vi "Banana_Equal Type Comparison.vi"(6 "verbose? (F)":bool, 7 "Not? (F)":bool, 8 "error in (no error)":errorcluster, 9 "Y":variant, 10 "X":variant) -> (0 "error out":errorcluster, 2 "Equal Types?":bool, 3 "Verbose output":string)   [LabVIEW 2021, in "Bananas.lvlib"]
uses:
  Bananas.lvlib
  <vilib>/Utility/VariantDataType/Type.ctl
  <vilib>/Utility/VariantDataType/VariantType.lvlib
  <vilib>/Utility/Data Type/NI_Data Type.lvlib
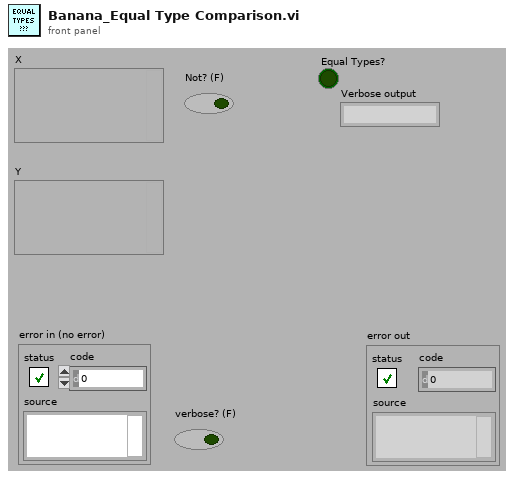
[diagram p1: front panel]
types:
  T1 = typedef "NI_Data Type.lvlib/Data Type.ctl" = enum8{"Invalid Type", "Void", "I8", "I16", "I32", "I64", "U8", "U16", "U32", "U64", "Single Float", "Double Float", "Extended Float", "Single Complex", "Double Complex", "Extended Complex", "Enum U8", "Enum U16", "Enum U32", "Enum U64", "Single Float With Unit", "Double Float With Unit", "Extended Float With Unit", "Single Complex with Unit", "Double Complex with Unit", "Extended Complex with Unit", "Boolean", "String", "Path", "Picture", "Tag", "Array", "Cluster", "Variant", "LV Variant", "Waveform", "Timestamp", "Digital Waveform", "Digital Data", "ExpressData", "Refnum", "External Data", "VI", "Poly VI", "LabVIEW Class Instance", "Fixed Point", "Set Collection", "Map Collection"}
  T2 = typedef "VariantType.lvlib/Type.ctl" = enum8{"Invalid Type", "Void", "I8", "I16", "I32", "I64", "U8", "U16", "U32", "U64", "Single Float", "Double Float", "Extended Float", "Single Complex", "Double Complex", "Extended Complex", "Enum U8", "Enum U16", "Enum U32", "Enum U64", "Single Float With Unit", "Double Float With Unit", "Extended Float With Unit", "Single Complex with Unit", "Double Complex with Unit", "Extended Complex with Unit", "Boolean", "String", "Path", "Picture", "Tag", "Array", "Cluster", "Variant", "LV Variant", "Waveform", "Timestamp", "Digital Waveform", "Digital Data", "ExpressData", "Refnum", "External Data", "VI", "Poly VI", "LabVIEW Class Instance", "Fixed Point"}
  T3 = typedef "NI_Data Type.lvlib/Refnum Type.ctl" = enum16{"NotARefnum", "UnknownRefnum", "Generic", "Datalog", "ByteStream", "Device", "Occurence", "TCPNetConnection", "Auto", "Menu", "Imaq", "Hardware", "DataSocket", "Visa", "IVI", "UDPNetConnection", "Notifier", "Queue", "Irda", "EventReg", "DotNet", "UserEvent", "Callback", "UNUSED_EMPTY_POSITION", "BlueToothNetConnection", "LVObjApp", "LVObjVI", "LVObjUnknown", "GenericClass", "UserDefinedRefnumTag", "DataValue", "RT FIFO", "TDMS File", "PythonSessionRefnum"}
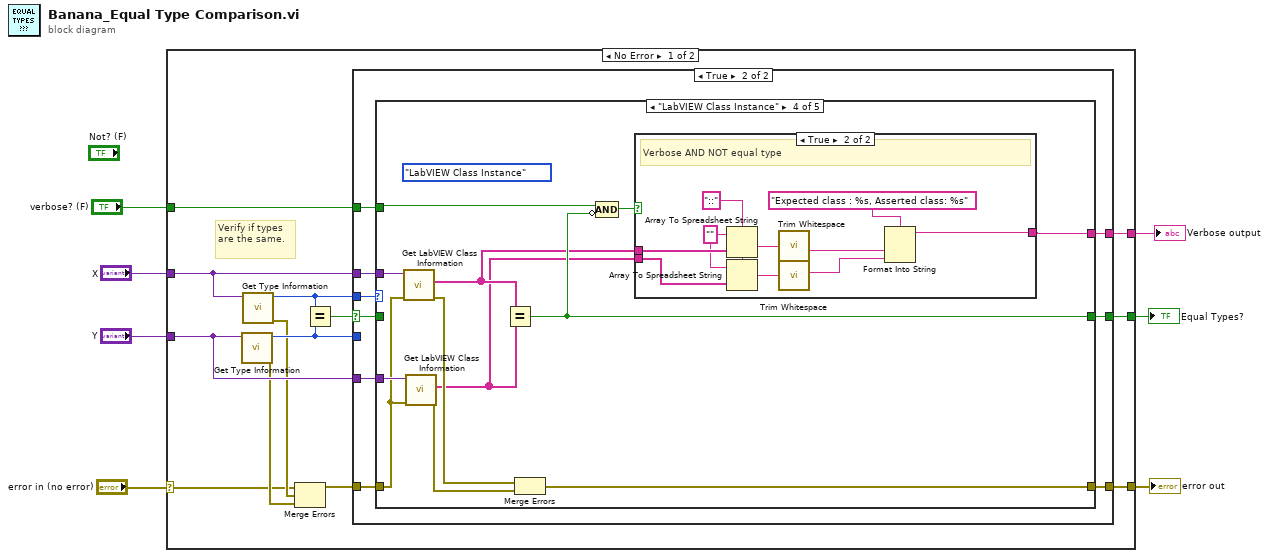
[diagram p0: block diagram]
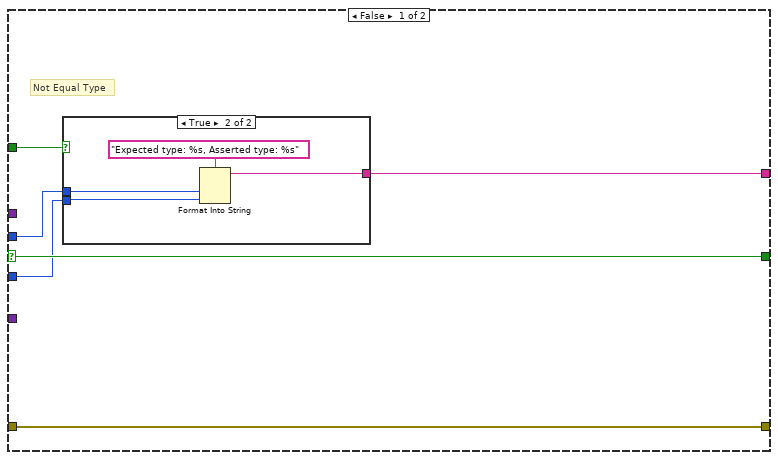
[diagram p2: hidden frame]
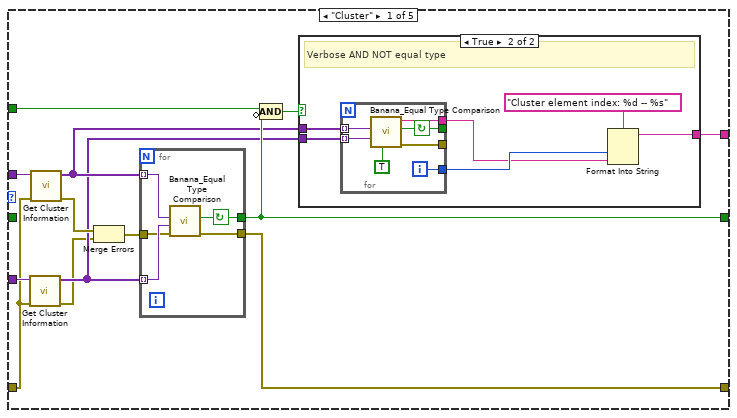
[diagram p4: hidden frame]
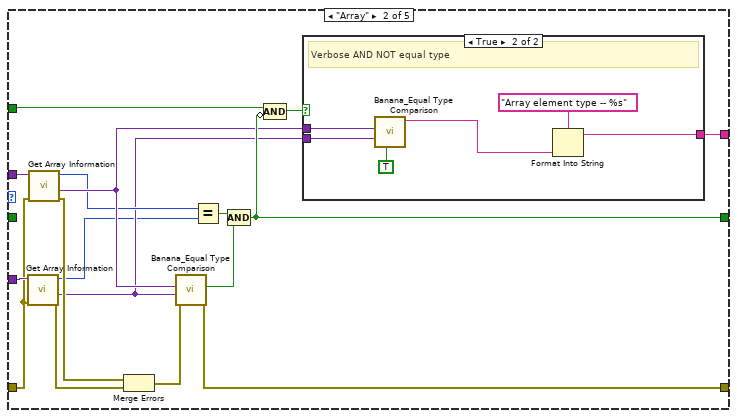
[diagram p6: hidden frame]
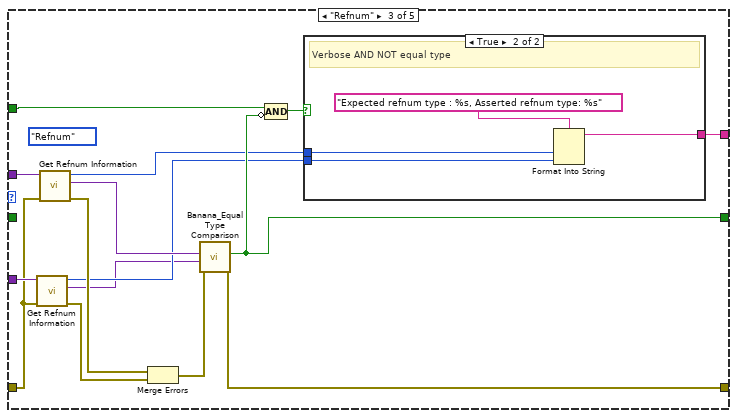
[diagram p8: hidden frame]
diagram:
  n1 = case shown="No Error" "error in (no error)" {
    selector: "error in (no error)" -> [w8 w137]
    tunnel: "X" -> [w14 _]
    tunnel: "Y" -> [w12 _]
    tunnel: [w18 w137] -> w7
    tunnel: [w17 _] -> w6
    tunnel: "verbose? (F)" -> [w16 _]
    tunnel: [w15 _] -> w4
    frame No Error {
      # "Verify if types are the same."
      n2 = call <vilib>:"Get Type Information.vi"("variant"=w12) -> ("error out"=w9:errorcluster, "type"=w11:T1)  [unwired: 6 in, 3 out]
      n3 = call <vilib>:"Get Type Information.vi"("variant"=w14) -> ("error out"=w10:errorcluster, "type"=w13:T1)  [unwired: 6 in, 3 out]
      n4 = Merge Errors(w8, w10, w9) -> (w19:errorcluster)
      n5 = Equal?(x=w13, y=w11) -> (x = y?=w20:bool)
      n6 = case shown="True" w20 {
        selector: w20 -> [w26 w38]
        tunnel: [w26 w37] -> w17
        tunnel: w13 -> [w24 w39]
        tunnel: w14 -> [_ w36]
        tunnel: w12 -> [_ w35]
        tunnel: w19 -> [w25 w34]
        tunnel: [w25 w33] -> w18
        tunnel: w11 -> [w22 _]
        tunnel: w16 -> [w23 w32]
        tunnel: [w21 w31] -> w15
        frame False {
          # "Not Equal Type"
          n7 = case shown="True" w23 {
            tunnel: w24 -> [_ w30]
            tunnel: w22 -> [_ w29]
            tunnel: [_ w27] -> w21
            frame False {
            }
            frame True {
              n8 = Format Into String(format string="Expected type: %s, Asserted type: %s", w30, w29) -> (resulting string=w27:string)  [unwired: 2 in, 1 out]
            }
          }
        }
        frame True {
          n9 = case shown="\"LabVIEW Class Instance\"" w39 {
            tunnel: [w48 w80 w103 w120 w136] -> w37
            tunnel: w38 -> [_ _ _ _ w136]
            tunnel: w36 -> [w46 w79 w101 w119 _]
            tunnel: w35 -> [w43 w75 w98 w116 _]
            tunnel: w34 -> [w42 w74 w97 w113 w135]
            tunnel: [w52 w84 w107 w124 w135] -> w33
            tunnel: w32 -> [w50 w81 w104 w121 _]
            tunnel: [w47 w83 w105 w122 _] -> w31
            frame "Cluster" {
              n10 = call <vilib>:"Get Cluster Information.vi"("error in (no error)"=w42, "variant"=w43) -> ("error out"=w40:errorcluster, "cluster elements"=w41:variant[])  [unwired: 8 in]
              n11 = call <vilib>:"Get Cluster Information.vi"("error in (no error)"=w42, "variant"=w46) -> ("error out"=w44:errorcluster, "cluster elements"=w45:variant[])  [unwired: 8 in]
              n12 = Merge Errors(w44, w40) -> (w51:errorcluster)
              n13 = for {
                tunnel: [w68] -> w48
                tunnel: w45 -> [w70] mode=indexing
                tunnel: w41 -> [w69] mode=indexing
                tunnel: w51 -> [w67]
                tunnel: [w66] -> w52
                stop <- w68 continue-if-true
                n14 = call "Banana_Equal Type Comparison.vi"("error in (no error)"=w67, "Y"=w69, "X"=w70) -> ("error out"=w66:errorcluster, "Equal Types?"=w68:bool)  [unwired: 6 in, 1 out]
              }
              n15 = Compound Arithmetic op=AND(w50, invert w48) -> (w49:bool)
              n16 = case shown="True" w49 {
                tunnel: w45 -> [_ w58]
                tunnel: w41 -> [_ w57]
                tunnel: [_ w56] -> w47
                frame False {
                }
                frame True {
                  # "Verbose AND NOT equal type"
                  n17 = for {
                    tunnel: [w63] -> _
                    tunnel: w58 -> [w65] mode=indexing
                    tunnel: w57 -> [w64] mode=indexing
                    tunnel: [w62] -> _
                    tunnel: [w60] -> w55
                    tunnel: [w59] -> w54
                    i -> [w60]
                    stop <- w63 continue-if-true
                    n18 = call "Banana_Equal Type Comparison.vi"("verbose? (F)"=TRUE, "Y"=w64, "X"=w65) -> ("error out"=w62:errorcluster, "Equal Types?"=w63:bool, "Verbose output"=w59:string)  [unwired: 6 in]
                  }
                  n19 = Format Into String(format string="Cluster element index: %d -- %s", w55, w54) -> (resulting string=w56:string)  [unwired: 2 in, 1 out]
                }
              }
            }
            frame "Array" {
              n20 = call <vilib>:"Get Array Information.vi"("error in (no error)"=w74, "variant"=w75) -> ("error out"=w73:errorcluster, "array element data type"=w72:variant, "number of dimensions"=w71:i32)  [unwired: 6 in, 1 out]
              n21 = call <vilib>:"Get Array Information.vi"("error in (no error)"=w74, "variant"=w79) -> ("error out"=w76:errorcluster, "array element data type"=w78:variant, "number of dimensions"=w77:i32)  [unwired: 6 in, 1 out]
              n22 = Merge Errors(w76, w73) -> (w85:errorcluster)
              n23 = call "Banana_Equal Type Comparison.vi"("error in (no error)"=w85, "Y"=w72, "X"=w78) -> ("error out"=w84:errorcluster, "Equal Types?"=w86:bool)  [unwired: 6 in, 1 out]
              n24 = Equal?(x=w77, y=w71) -> (x = y?=w87:bool)
              n25 = Compound Arithmetic op=AND(w87, w86) -> (w80:bool)
              n26 = Compound Arithmetic op=AND(w81, invert w80) -> (w82:bool)
              n27 = case shown="True" w82 {
                tunnel: w78 -> [_ w93]
                tunnel: w72 -> [_ w92]
                tunnel: [_ w91] -> w83
                frame False {
                }
                frame True {
                  # "Verbose AND NOT equal type"
                  n28 = call "Banana_Equal Type Comparison.vi"("verbose? (F)"=TRUE, "Y"=w92, "X"=w93) -> ("Verbose output"=w90:string)  [unwired: 6 in, 2 out]
                  n29 = Format Into String(format string="Array element type -- %s", w90) -> (resulting string=w91:string)  [unwired: 2 in, 1 out]
                }
              }
            }
            frame "Refnum" {
              (unwired) Type."Refnum" ("Type Enum")
              n30 = call <vilib>:"Get Refnum Information.vi"("error in (no error)"=w97, "variant"=w98) -> ("error out"=w94:errorcluster, "strict type"=w95:variant, "reference type"=w96:T3)  [unwired: 6 in, 1 out]
              n31 = call <vilib>:"Get Refnum Information.vi"("error in (no error)"=w97, "variant"=w101) -> ("error out"=w99:errorcluster, "strict type"=w102:variant, "reference type"=w100:T3)  [unwired: 6 in, 1 out]
              n32 = Merge Errors(w99, w94) -> (w108:errorcluster)
              n33 = call "Banana_Equal Type Comparison.vi"("error in (no error)"=w108, "Y"=w95, "X"=w102) -> ("error out"=w107:errorcluster, "Equal Types?"=w103:bool)  [unwired: 6 in, 1 out]
              n34 = Compound Arithmetic op=AND(w104, invert w103) -> (w106:bool)
              n35 = case shown="True" w106 {
                tunnel: [_ w112] -> w105
                tunnel: w100 -> [_ w110]
                tunnel: w96 -> [_ w109]
                frame False {
                }
                frame True {
                  # "Verbose AND NOT equal type"
                  n36 = Format Into String(format string="Expected refnum type : %s, Asserted refnum type: %s", w110, w109) -> (resulting string=w112:string)  [unwired: 2 in, 1 out]
                }
              }
            }
            frame "LabVIEW Class Instance" {
              (unwired) Type."LabVIEW Class Instance" ("Type Enum")
              n37 = call <vilib>:"Get LabVIEW Class Information.vi"("error in (no error)"=w113, "variant"=w119) -> ("error out"=w117:errorcluster, "qualified LabVIEW class name"=w118:string[])  [unwired: 7 in, 1 out]
              n38 = call <vilib>:"Get LabVIEW Class Information.vi"("error in (no error)"=w113, "variant"=w116) -> ("error out"=w114:errorcluster, "qualified LabVIEW class name"=w115:string[])  [unwired: 7 in, 1 out]
              n39 = Equal?(x=w118, y=w115) -> (x = y?=w120:bool)
              n40 = Merge Errors(w117, w114) -> (w124:errorcluster)
              n41 = Compound Arithmetic op=AND(w121, invert w120) -> (w123:bool)
              n42 = case shown="True" w123 {
                tunnel: [_ w134] -> w122
                tunnel: w118 -> [_ w131]
                tunnel: w115 -> [_ w133]
                frame False {
                }
                frame True {
                  w125 = "::" ("delimiter (Tab)")
                  w126 = "" ("format string")
                  # "Verbose AND NOT equal type"
                  n43 = Array To Spreadsheet String(delimiter (Tab)=w125, array=w131, 3:w126) -> (spreadsheet string=w130:string)
                  n44 = Array To Spreadsheet String(delimiter (Tab)=w125, array=w133, 3:w126) -> (spreadsheet string=w129:string)
                  n45 = call <vilib>:"Trim Whitespace.vi"("string"=w130) -> ("trimmed string"=w128:string)  [unwired: 1 in]
                  n46 = call <vilib>:"Trim Whitespace.vi"("string"=w129) -> ("trimmed string"=w127:string)  [unwired: 1 in]
                  n47 = Format Into String(format string="Expected class : %s, Asserted class: %s", w128, w127) -> (resulting string=w134:string)  [unwired: 2 in, 1 out]
                }
              }
            }
            frame Default {
            }
          }
        }
      }
    }
    frame Error {
    }
  }
  "Equal Types?" <- w6
  "error out" <- w7
  "Verbose output" <- w4
